vi "example test.vi"() -> ()   [LabVIEW 2013, in "tdms logger tests.lvlib"]
uses:
  tdms logger tests.lvlib
  <vilib>/NI/Tag Bus/tag/Data Type.ctl
  <vilib>/NI/Tag Bus Module Framework/channel/channel classification.ctl
  configuration/TDMS datalogger configuration.lvclass
  execution/TDMS datalogger runtime.lvclass
  configuration/TDMS datalogger configuration.lvclass/TDMS datalogger configuration.ctl
  <vilib>/NI/Tag Bus/dictionary/data dictionary.lvclass/data dictionary.ctl
  <vilib>/NI/Tag Bus/dictionary/lookup polymorphs/locate double.vi
  <vilib>/NI/Tag Bus/table/data polymorphs/write one/write Double.vi
  configuration/Write channels.vi
  configuration/Write backup directory.vi
  configuration/Write Path.vi
  <vilib>/NI/Tag Bus/dictionary/search/find data index.vi
  <vilib>/NI/Tag Bus/dictionary/search/search string list.vi
  <vilib>/NI/Tag Bus/dictionary/tag not found.vi
  <vilib>/NI/Tag Bus Module Framework/channel/TBM channel.lvclass
  <vilib>/NI/Tag Bus/tag/tag descriptor.lvclass
  <vilib>/NI/Tag Bus/dictionary/data dictionary.lvclass
  <vilib>/NI/Tag Bus/table/data table.lvlib
panel:
  out "final error":errorcluster
  out "output error":errorcluster
  out "output lookup error":errorcluster
  out "init error":errorcluster
  out "correct execution settings":bool
  out "serialization problem":errorcluster
  out "invalid configuration":errorcluster
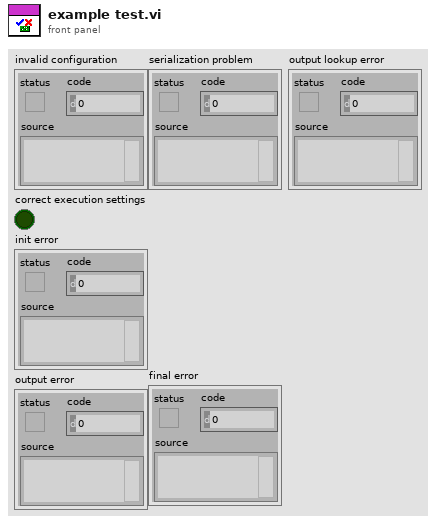
[diagram p1: front panel]
types:
  T1 = typedef "TBM channel.lvclass/channel classification.ctl" = enum16{"input data", "output data", "processing parameter", "processing result"}
  T2 = typedef "tag bus.lvlib/tag descriptor.lvclass/Data Type.ctl" = enum16{"Double", "Single", "I64", "I32", "I16", "I8", "U64", "U32", "U16", "U8", "Boolean", "String", "Array of Double", "Array of Single", "Array of I64", "Array of I32", "Array of I16", "Array of I8", "Array of U64", "Array of U32", "Array of U16", "Array of U8", "Array of Boolean", "Array of String"}
  T3 = typedef "TBM channel.lvclass/data tables.ctl" = cluster{"input data":T4, "processing parameter":T4, "processing result":T4, "output data":T4}
  T4 = typedef "tag bus.lvlib/dictionary table pair.ctl" = cluster{"data dictionary":refnum<class "data dictionary.lvclass">, "data table":T5}
  T5 = typedef "tag bus.lvlib/data table.lvlib/data table.ctl" = cluster{"Double":dbl[], "Single":sgl[], "I64":i64[], "I32":i32[], "I16":i16[], "I8":i8[], "U64":u64[], "U32":u32[], "U16":u16[], "U8":u8[], "Boolean":bool[], "String":string[], "Array of Double":cluster{"DBL Array":dbl[]}[], "Array of Single":cluster{"SGL Array":sgl[]}[], "Array of I64":cluster{"I64 Array":i64[]}[], "Array of I32":cluster{"I32 Array":i32[]}[], "Array of I16":cluster{"I16 Array":i16[]}[], "Array of I8":cluster{"I8 Array":i8[]}[], "Array of U64":cluster{"U64 Array":u64[]}[], "Array of U32":cluster{"U32 Array":u32[]}[], "Array of U16":cluster{"U16 Array":u16[]}[], "Array of U8":cluster{"U8 Array":u8[]}[], "Array of Boolean":cluster{"Boolean Array":bool[]}[], "Array of String":cluster{"String Array":string[]}[]}
  T6 = typedef "TBM module execution interface.lvclass/execution settings.ctl" = cluster{"reads inputs":bool, "processes data":bool, "writes outputs":bool}
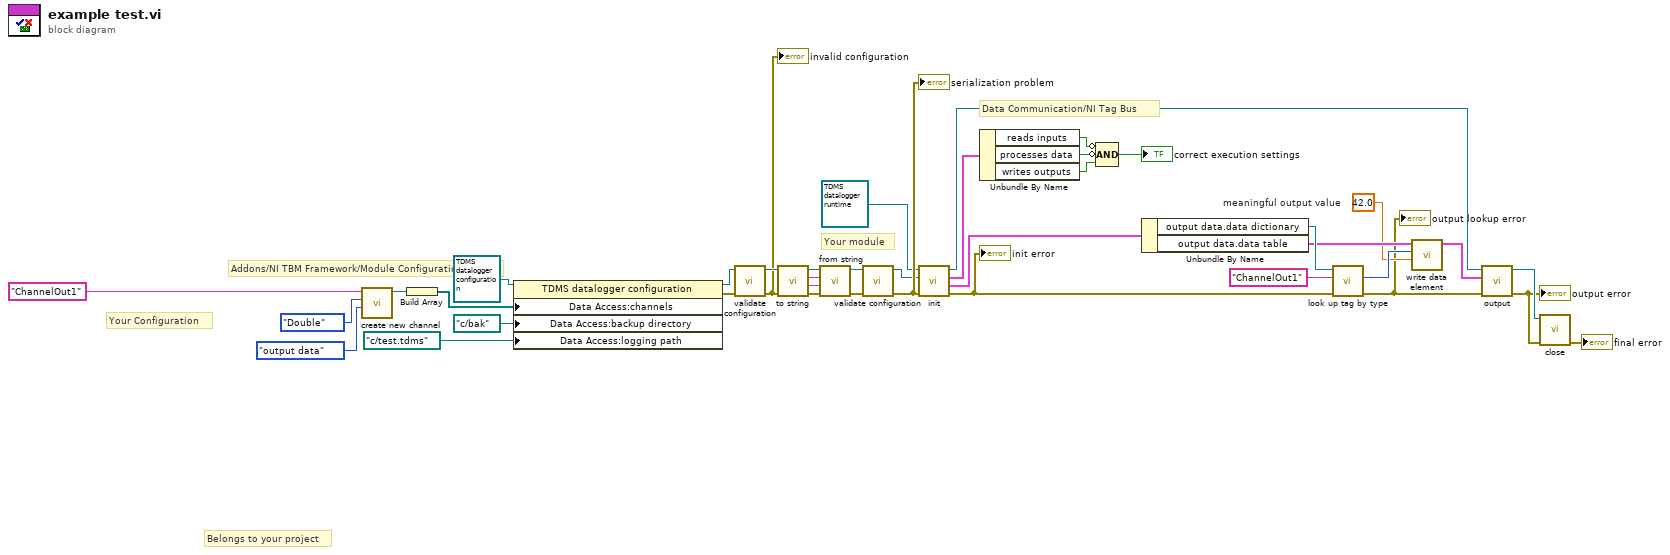
[diagram p0: block diagram]
diagram:
  w14 = 42.0  # meaningful output value
  # "Data Communication/NI Tag Bus"
  # "Your module"
  # "Your Configuration"
  # "Addons/NI TBM Framework/Module Configuration"
  # "Belongs to your project"
  n1 = call <vilib>:"create new channel.vi"("channel classification"=channel_classification."output data", "data type"=Data_Type."Double", "channel name"="ChannelOut1") -> ("channel"=w8:refnum<class "TBM channel.lvclass">)  [unwired: 8 in]
  n2 = Build Array(w8) -> (w5:refnum<class "TBM channel.lvclass">[])
  n3 = property class="TDMS datalogger configuration"(reference=refnum<class "TDMS datalogger configuration.lvclass"> refnum ("TDMS datalogger configuration"), "Data Access:channels"=w5, "Data Access:backup directory"=path "c:/bak" ("backup directory"), "Data Access:logging path"=path "c:/test.tdms" ("logging path")) -> (reference out=w7:refnum<class "TDMS datalogger configuration.lvclass">, error out=w6:errorcluster)  [unwired: 1 in]
  n4 = call-dynamic "validate configuration.vi"("error in"=w6, "TDMS datalogger configuration in"=w7) -> ("error out"=w35:errorcluster, "TDMS datalogger configuration out"=w36:refnum<class "TDMS datalogger configuration.lvclass">)  [unwired: 8 in]
  "invalid configuration" <- w35
  n5 = call-dynamic "to string.vi"("error in"=w35, "TDMS datalogger configuration in"=w36) -> ("error out"=w31:errorcluster, "data"=w32:string, "version"=w33:string, "TDMS datalogger configuration out"=w34:refnum<class "TDMS datalogger configuration.lvclass">)  [unwired: 6 in]
  n6 = call-dynamic "from string.vi"("error in"=w31, "data"=w32, "version"=w33, "TDMS datalogger configuration in"=w34) -> ("error out"=w29:errorcluster, "TDMS datalogger configuration out"=w30:refnum<class "TDMS datalogger configuration.lvclass">)  [unwired: 6 in]
  n7 = call-dynamic "validate configuration.vi"("error in"=w29, "TDMS datalogger configuration in"=w30) -> ("error out"=w28:errorcluster, "TDMS datalogger configuration out"=w27:refnum<class "TDMS datalogger configuration.lvclass">)  [unwired: 8 in]
  "serialization problem" <- w28
  n8 = call-dynamic "init.vi"("error in"=w28, "TBM module configuration in"=w27, "TDMS datalogger runtime in"=refnum<class "TDMS datalogger runtime.lvclass"> refnum ("TDMS datalogger runtime")) -> ("error out"=w20:errorcluster, "data allocations"=w21:T3, "execution settings"=w26:T6, "TDMS datalogger runtime out"=w19:refnum<class "TDMS datalogger runtime.lvclass">)  [unwired: 5 in]
  "init error" <- w20
  n9 = Unbundle By Name(w26) -> ("reads inputs"=w23:bool, "processes data"=w25:bool, "writes outputs"=w24:bool)
  n10 = Compound Arithmetic op=AND(invert w23, invert w25, w24) -> (→"correct execution settings":bool)
  n11 = Unbundle By Name(w21) -> ("output data.data dictionary"=w18:refnum<class "data dictionary.lvclass">, "output data.data table"=w15:T5)
  n12 = call-poly <vilib>:"look up tag by type.vi"("error in"=w20, "name"="ChannelOut1" ("channel name"), "data dictionary in"=w18) -> ("error out"=w13:errorcluster, "index"=w16:i32)  [unwired: 6 in, 1 out]
  "output lookup error" <- w13
  n13 = call-poly <vilib>:"write data element.vi"("value"=w14, "index"=w16, "data table in"=w15) -> ("data table out"=w12:T5)  [unwired: 8 in]
  n14 = call-dynamic "output.vi"("error in"=w13, "data table in"=w12, "TDMS datalogger runtime in"=w19) -> ("error out"=w10:errorcluster, "TDMS datalogger runtime out"=w11:refnum<class "TDMS datalogger runtime.lvclass">)  [unwired: 6 in, 1 out]
  "output error" <- w10
  n15 = call-dynamic "close.vi"("error in"=w10, "TDMS datalogger runtime in"=w11) -> ("error out"=→"final error":errorcluster)  [unwired: 9 in]
